vi "WillDey_Demux.vi"() -> ()   [LabVIEW 2017]
panel:
  in  "stop":bool
  in  "milliseconds to wait":u32
  in  "Card Slot 2":i8
  in  "VISA resource name":refnum<visa-resource-name>
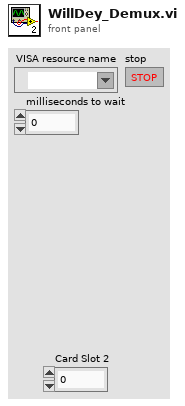
[diagram p1: front panel]
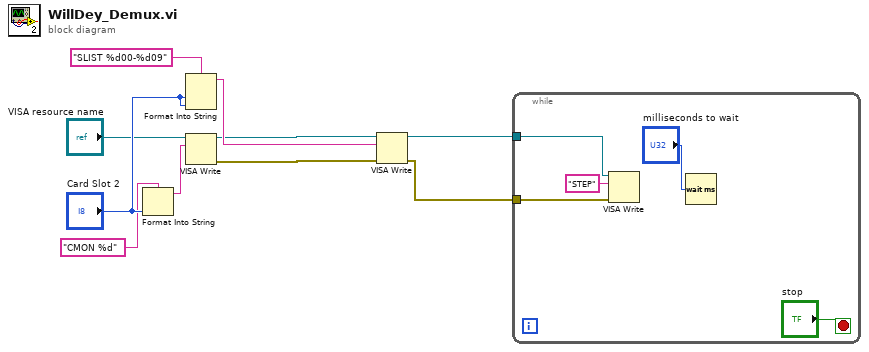
[diagram p0: block diagram]
diagram:
  n1 = Format Into String(format string="CMON %d" ("write buffer"), "Card Slot 2") -> (resulting string=w6:string)  [unwired: 2 in, 1 out]
  n2 = Format Into String(format string="SLIST %d00-%d09" ("write buffer"), "Card Slot 2", "Card Slot 2") -> (resulting string=w9:string)  [unwired: 2 in, 1 out]
  n3 = VISA Write(VISA resource name="VISA resource name", write buffer=w6) -> (VISA resource name out=w4:refnum<visa-resource-name>, error out=w3:errorcluster)  [unwired: 1 in, 1 out]
  n4 = VISA Write(VISA resource name=w4, write buffer=w9, error in (no error)=w3) -> (VISA resource name out=w2:refnum<visa-resource-name>, error out=w1:errorcluster)  [unwired: 1 out]
  n5 = while {
    tunnel: w2 -> [w14]
    tunnel: w1 -> [w13]
    stop <- "stop" stop-if-true
    n6 = VISA Write(VISA resource name=w14, write buffer="STEP", error in (no error)=w13) -> ()  [unwired: 3 out]
    n7 = Wait (ms)(milliseconds to wait="milliseconds to wait") -> ()  [unwired: 1 out]
  }
